vi "Create 9759.vi"(8 "error in (no error)":errorcluster, 11 "Section Ptr":T1 format="%.0x") -> (0 "error out":errorcluster, 3 "Section Ptr dup":T1 format="%.0x")   [LabVIEW 2015, in "NI 9759 RevB Custom Device.lvlib"]
uses:
  NI 9759 RevB Custom Device.lvlib
  <vilib>/NI Veristand/Custom Device API/Custom Device Item Ref.ctl
  <vilib>/NI Veristand/Custom Device API/Custom Device Channel Type.ctl
  Shared/9759 Constants and GUIDs.vi
  <vilib>/NI VeriStand/Custom Device API/Custom Device API.lvlib
  <vilib>/NI Veristand/Custom Device Tools/Custom Device Utility Library/Custom Device Utility Library.lvlib
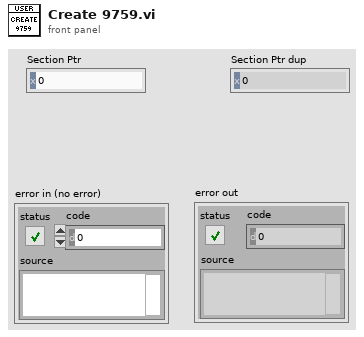
[diagram p1: front panel]
types:
  T1 = typedef "Custom Device API.lvlib/Custom Device Item Ref.ctl" = u64
  T2 = typedef "Custom Device API.lvlib/Custom Device Channel Type.ctl" = enum16{"Input", "Output"}
  T3 = typedef "NI 9759 RevB Custom Device.lvlib/Channel.ctl" = cluster{"Name":string, "Units":string, "Default":dbl, "Description":string}
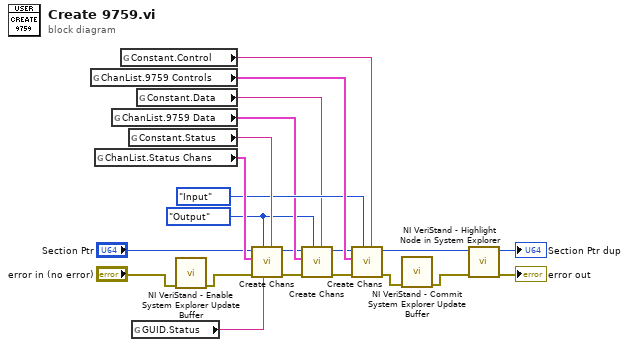
[diagram p0: block diagram]
diagram:
  w3 = Custom_Device_Channel_Type."Output" ("Type")
  n1 = global read "9759 Constants and GUIDs.vi" "ChanList.9759 Controls"() -> (w14:T3[])
  n2 = global read "9759 Constants and GUIDs.vi" "ChanList.Status Chans"() -> (w16:T3[])
  n3 = global read "9759 Constants and GUIDs.vi" "ChanList.9759 Data"() -> (w10:T3[])
  n4 = global read "9759 Constants and GUIDs.vi" "Constant.Control"() -> (w13:string)
  n5 = global read "9759 Constants and GUIDs.vi" "Constant.Status"() -> (w17:string)
  n6 = global read "9759 Constants and GUIDs.vi" "GUID.Status"() -> (w15:string)
  n7 = global read "9759 Constants and GUIDs.vi" "Constant.Data"() -> (w11:string)
  n8 = call <vilib>:"NI VeriStand - Enable System Explorer Update Buffer.vi"("error in (no error)"="error in (no error)") -> ("error out"=w2:errorcluster)  [unwired: 10 in]
  n9 = call "Create Chans.vi"("New Section Name (none)"=w17, "new section GUID (\"\":del prot)"=w15, "Type"=w3, "error in (no error)"=w2, "Channels"=w16, "Section Ptr"="Section Ptr") -> ("error out"=w6:errorcluster, "Section Ptr dup"=w7:T1)  [unwired: 2 in, 2 out]
  n10 = call "Create Chans.vi"("New Section Name (none)"=w11, "Type"=w3, "error in (no error)"=w6, "Channels"=w10, "Section Ptr"=w7) -> ("error out"=w5:errorcluster, "Section Ptr dup"=w4:T1)  [unwired: 3 in, 2 out]
  n11 = call "Create Chans.vi"("New Section Name (none)"=w13, "Type"=Custom_Device_Channel_Type."Input", "error in (no error)"=w5, "Channels"=w14, "Section Ptr"=w4) -> ("error out"=w9:errorcluster, "Section Ptr dup"=w8:T1)  [unwired: 3 in, 2 out]
  n12 = call <vilib>:"NI VeriStand - Commit System Explorer Update Buffer.vi"("error in (no error)"=w9) -> ("error out"=w20:errorcluster)  [unwired: 10 in]
  n13 = call <vilib>:"NI VeriStand - Highlight Node in System Explorer.vi"("error in (no error)"=w20, "Item Ref in"=w8) -> ("error out"=→"error out":errorcluster, "Node Ptr dup"=→"Section Ptr dup":T1)  [unwired: 8 in]
